vi "RM.getReservationListStrings.vi"(8 "error in":errorcluster, 9 "ClientInfo Array":T1[](array[typedef]) {"CD Ref" format="%.0x"}, 10 "type filter":i32=-1, 11 "reservation db":variant) -> (0 "error out":errorcluster, 3 "Reservation List Array":string[][](array[string]))   [LabVIEW 2016, in "FPGA Resource Manager.lvlib"]
uses:
  FPGA Resource Manager.lvlib
  RM.clientInfo.ctl
  <vilib>/NI Veristand/Custom Device API/Custom Device Item Ref.ctl
  <vilib>/NI Veristand/Custom Device API/Custom Device API.lvlib
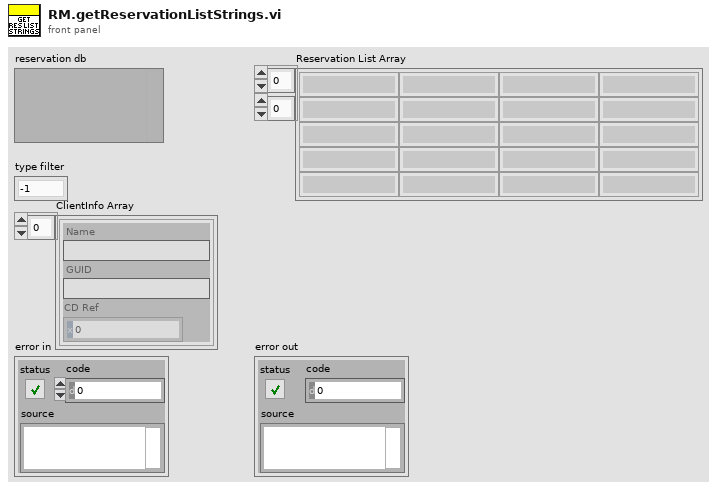
[diagram p1: front panel]
types:
  T1 = typedef "FPGA Resource Manager.lvlib/RM.clientInfo.ctl" = cluster{"Name":string, "GUID":string, "CD Ref":T2}
  T2 = typedef "Custom Device API.lvlib/Custom Device Item Ref.ctl" = u64
  T3 = typedef "FPGA Resource Manager.lvlib/RM.resourceType.ctl" = enum16{"Scalar Input", "Scalar Output", "Waveform Input", "Waveform Output"}
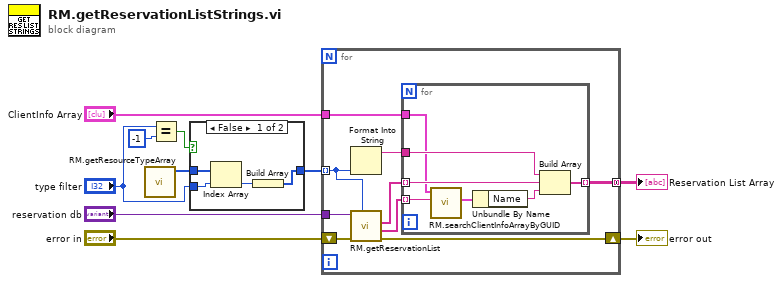
[diagram p0: block diagram]
diagram:
  n1 = call "RM.getResourceTypeArray.vi"() -> ("Array"=w4:T3[])  [unwired: 11 in]
  n2 = Equal?(x="type filter", y=-1) -> (x = y?=w5:bool)
  n3 = case shown="False" w5 {
    tunnel: w4 -> [w14 w15]
    tunnel: [w11 w15] -> w3
    tunnel: "type filter" -> [w12 _]
    frame False {
      n4 = Index Array(array=w14, index=w12) -> (element=w13:T3)
      n5 = Build Array(w13) -> (w11:T3[])
    }
    frame True {
    }
  }
  n6 = for {
    tunnel: [w17] -> w7 mode=concatenating
    tunnel: "reservation db" -> [w24]
    tunnel: w3 -> [w21] mode=indexing
    shift-right: [w22] -> w8
    shift-left: "error in" -> [w23]
    tunnel: "ClientInfo Array" -> [w16]
    n7 = Format Into String(w21) -> (resulting string=w18:string)  [unwired: 3 in, 1 out]
    n8 = call "RM.getReservationList.vi"("Resource Type"=w21, "error in"=w23, "reservation DB in"=w24) -> ("error out"=w22:errorcluster, "clientGUIDs"=w19:string[], "names in bitfile"=w20:string[])  [unwired: 5 in, 1 out]
    n9 = for {
      tunnel: w20 -> [w30] mode=indexing
      tunnel: w19 -> [w28] mode=indexing
      tunnel: w18 -> [w31]
      tunnel: [w29] -> w17 mode=indexing
      tunnel: w16 -> [w27]
      n10 = call "RM.searchClientInfoArrayByGUID.vi"("ClientGUID"=w28, "Client Array in"=w27) -> ("ClientInfo"=w26:T1)  [unwired: 6 in, 3 out]
      n11 = Unbundle By Name(w26) -> ("Name"=w25:string)
      n12 = Build Array(w31, w30, w25) -> (w29:string[])
    }
  }
  "Reservation List Array" <- w7
  "error out" <- w8
